vi "Consumer.vi"(8 "error in (no error)":errorcluster, 9 "Data":variant, 10 "Case ID":string, 11 "uService Template in":refnum<class "DAQ Sender.lvclass">) -> (0 "error out":errorcluster, 3 "uService Template out":refnum<class "DAQ Sender.lvclass">)   [LabVIEW 2020, in "DAQ Sender.lvlib" / "DAQ Sender.lvclass"]
uses:
  DAQ Sender.lvclass
  DAQ Sender Consumer Case Selector.ctl
  TALOS/TALOS_PPL.lvlibp/Interfaces/DAQ Communication/DAQ Message.ctl
  DAQ Sender.lvclass/DAQ Sender.ctl
  TALOS/TALOS_PPL.lvlibp/Father of all uServices/Father of all uServices/Father of all uServices.lvclass
  TALOS/TALOS_PPL.lvlibp
  TALOS/TALOS_PPL.lvlibp/Interfaces/DAQ Communication/DAQ Communication.lvclass
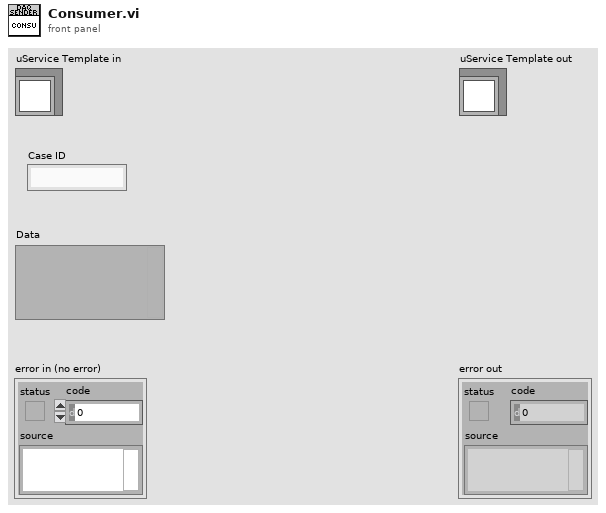
[diagram p1: front panel]
types:
  T1 = typedef "DAQ Sender.lvlib/DAQ Sender.lvclass/DAQ Sender Consumer Case Selector.ctl" = enum16{"Send to DAQ"}
  T2 = typedef "TALOS_PPL.lvlibp/Interfaces.lvlib/DAQ Communication.lvclass/DAQ Message.ctl" = cluster{"Path":string, "Port":u16, "Data Name":string, "Data":variant, "File?":bool, "Timestamp":timestamp}
  T3 = cluster{"Data":variant, "DAQ Address":cluster{"Port":u16, "Path":string}}
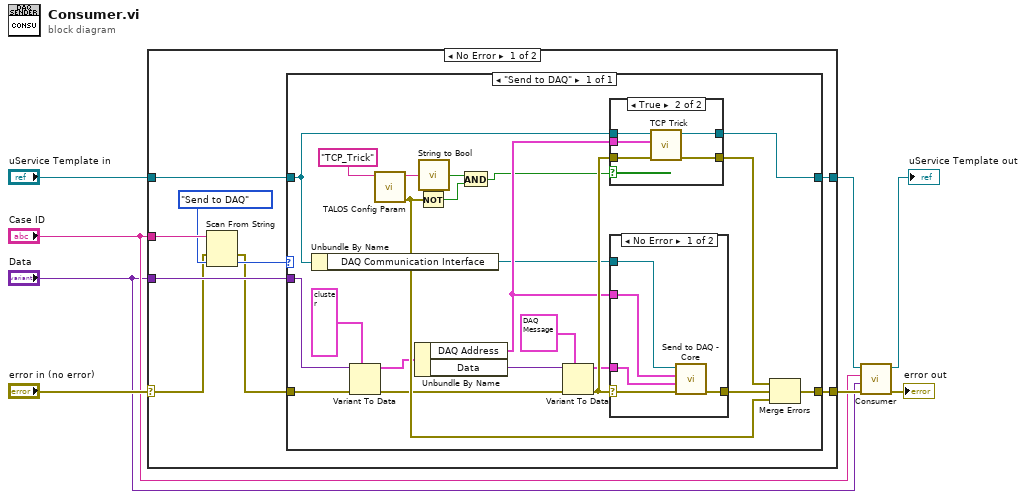
[diagram p0: block diagram]
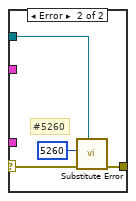
[diagram p3: hidden frame]
diagram:
  n1 = case shown="No Error" "error in (no error)" {
    selector: "error in (no error)" -> [w10 w56]
    tunnel: "uService Template in" -> [w16 w57]
    tunnel: [w14 w57] -> w4
    tunnel: [w15 w56] -> w3
    tunnel: "Case ID" -> [w13 _]
    tunnel: "Data" -> [w17 _]
    frame No Error {
      n2 = Scan From String(input string=w13, error in=w10, default 1=DAQ_Sender_Consumer_Case_Selector."Send to DAQ") -> (error out=w9:errorcluster, output 1=w11:T1)  [unwired: 2 in, 2 out]
      n3 = case shown="\"Send to DAQ\"" w11 {
        tunnel: w17 -> [w35]
        tunnel: w9 -> [w34]
        tunnel: w16 -> [w20]
        tunnel: [w22] -> w15
        tunnel: [w28] -> w14
        frame "Send to DAQ" {
          n4 = Unbundle By Name(w20) -> ("DAQ Communication Interface"=w19:refnum<class "DAQ Communication.lvclass">)
          n5 = Variant To Data(error in=w34, type=T3 {"Data"=variant, "DAQ Address"={"Port"=0, "Path"=""}} ("output cluster"), Variant=w35) -> (data=w32:T3, error out=w30:errorcluster)
          n6 = call "TALOS Config Param.vi"("Parameter Name"="TCP_Trick") -> ("error out"=w38:errorcluster, "Output"=w27:string)  [unwired: 9 in]
          n7 = Unbundle By Name(w32) -> ("DAQ Address"=w29:cluster{"Port":u16, "Path":string}, "Data"=w31:variant)
          n8 = Not(x=w38) -> (.not. x?=w24:bool)
          n9 = call "String to Bool.vi"("String"=w27) -> ("Boolean"=w25:bool)
          n10 = And(x=w25, y=w24) -> (x .and. y?=w23:bool)
          n11 = Variant To Data(error in=w30, type=T2 {"Path"="", "Port"=0, "Data Name"="", "Data"=variant, "File?"=FALSE, "Timestamp"=timestamp(0 s since 1904-01-01)} ("DAQ Message"), Variant=w31) -> (data=w37:T2, error out=w39:errorcluster)
          n12 = case shown="True" w23 {
            tunnel: w29 -> [_ w46]
            tunnel: [w41 w45] -> w28
            tunnel: w20 -> [w41 w44]
            tunnel: w39 -> [w40 w43]
            tunnel: [w40 w42] -> w21
            frame False {
            }
            frame True {
              n13 = call-dynamic "TCP Trick.vi"("error in (no error)"=w43, "DAQ Address"=w46, "DAQ Sender in"=w44) -> ("error out"=w42:errorcluster, "DAQ Sender out"=w45:refnum<class "DAQ Sender.lvclass">)  [unwired: 7 in]
            }
          }
          n14 = case shown="No Error" w39 {
            selector: w39 -> [w51 w54]
            tunnel: w37 -> [w47 _]
            tunnel: w19 -> [w49 w53]
            tunnel: [w50 w52] -> w36
            tunnel: w29 -> [w48 _]
            frame No Error {
              n15 = call "Send to DAQ - Core.vi"("error in (no error)"=w51, "DAQ Message"=w47, "DAQ Address"=w48, "DAQ Communication"=w49) -> ("error out"=w50:errorcluster)  [unwired: 7 in]
            }
            frame Error {
              # "#5260"
              n16 = call "Substitute Error.vi"("LabVIEW Object"=w53, "error in (no error)"=w54, "Error Code"=5260) -> ("error out"=w52:errorcluster)  [unwired: 8 in]
            }
          }
          n17 = Merge Errors(w21, w36, w38) -> (w22:errorcluster)
        }
      }
    }
    frame Error {
    }
  }
  n18 = call-parent "Consumer.vi"("error in (no error)"=w3, "Data"="Data", "Case ID"="Case ID", "uService Template in"=w4) -> ("error out"=→"error out":errorcluster, "uService Template out"=→"uService Template out":refnum<class "DAQ Sender.lvclass">)  [unwired: 6 in]
